vi "AlliGator Compute Phasor Plot's Phasor Ratio.vi"(4 "State Indicators Refnum":refnum<vi>, 5 "Time Stamp Array":dbl[](array[numeric]), 7 "Phasor Graph":refnum<vi>, 8 "Error In":errorcluster, 9 "Plot Idx":i32, 10 "Phasor Ratio Graph":refnum<vi>, 11 "Lifetime Graph":refnum<vi>) -> (0 "Error Out":errorcluster, 1 "Message":string)   [LabVIEW 2021, in "AlliGator Phasor Ratio.lvlib"]
doc: "Computes phasor ratio and derived quantities and outputs the corresponding plots."
uses:
  AlliGator Phasor Ratio.lvlib
  GUI/AlliGator State Indicator.ctl
  Settings/AlliGator Settings List.ctl
  Phasor/Phasor Ratio Type.ctl
  Phasor/Phasor.lvlib
  Globals, Variables, Constants/AlliGator Globals, Variables & Constants.lvlib
  Settings/AlliGator Settings.lvlib
  Graphs/XY Graph/XY Graph Add-Ons.lvlib
  Error/Error.lvlib
  Strings/Strings.lvlib
  Sound/Sound.lvlib
  GUI/AlliGator GUI.lvlib
panel:
  # "see the AlliGator License on the block diagram (Ctrl+E or Window:Show Block Diagram)"
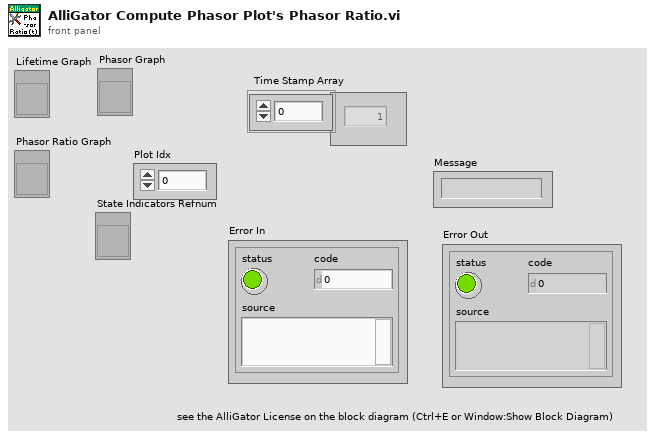
[diagram p1: front panel]
types:
  T1 = typedef "AlliGator State Indicator.ctl" = cluster{"Phasor Calibration Defined":bool, "Phasor Calibration Series Defined":bool, "Phasor Calibration Map Defined":bool, "Phasor Ratio Reference 1 Defined":bool, "Phasor Ratio Reference 2 Defined":bool, "Phasor Ratio Lifetime Reference 1 Defined ":bool, "Phasor Ratio Lifetime Reference 2 Defined":bool, "Phasor Calibration Used":bool, "Phasor Calibration Series Used":bool, "Phasor Calibration Map Used":bool, "Dataset Update Needed":bool, "Phasor Plot Update Needed":bool, "Reference/IRF Defined":bool, "Individual IRFs Defined":bool}
  T2 = typedef "AlliGator Settings.lvlib/AlliGator Settings List.ctl" = enum16{"GUI:Visible Settings Tab", "GUI:Last Run Version", "Source Image:Use Image Histogram for Contrast", "Source Image:Low Count Pixels Rejection Options", "Source Image:High Count Pixels Rejection Options", "Source Image:Use Image Brightness", "Source Image:Blend Overlay with Image Background", "Source Image:Use Fixed ROI Diameter", "Source Image:ROI Diameter", "Source Image:ROI Center Color", "Source Image:Peak Threshold", "Source Image:Intensity Threshold", "Source Image:Image Binning Options", "Source Image:Image Smoothing Options", "Source Image:Image Histogram Active", "Source Image:Invert Binary Mask", "Source Image:Hot Pixel Removal", "Source Image:Overlay Analyzed ROI Center", "Source Image:Auto-Adjust Contrast", "Source Image:Histogram Lower Percentile", "Source Image:Histogram Upper Percentile", "Source Image:Save Source Image", "Source Image:Scale Bar Options", "Source Image:Image Resolution (Pixel Size)", "Source Image:Flatfield Correction", "Source Image:Show Dead Left Columns Correction", "Source Image:Dead Left Columns Correction", "Source Image:Image Pre-Processing Operations Order", "Source Image:Overlay ROI Median", "Source Image:Median Overlay Color", "Data Information:Gate Width", "Data Information:Nanotime Gate Separation", "Data Information:Macrotime Gate Separation", "Data Information:Gate Step", "Data Information:# Gates", "Data Information:Gate Image Exposure", "Data Information:Gate Image Integration", "Data Information:Gates to Skip", "Data Information:Gates to Keep", "Data Information:Define Gates to", "Data Information:Channel Name", "Data Information:Available Channel Names", "Data Information:Channel Arithmetic", "Data Information:Background File Subtraction", "Data Information:Background File", "Data Information:Background Scaling Factor", "Data Information:Background Pile-up Correction", "Data Information:Background Pixel Well Capacity", "Data Information:Laser Period", "Data Information:SYNC Period", "Data Information:Pile-up Correction", "Data Information:Pixel Well Capacity", "Data Information:Dataset Scaling Factor", "Fluorescence Decay_Decay Pre-Processing:Reverse Gates", "Fluorescence Decay_Decay Pre-Processing:Verbose Decay Pre-Processing", "Fluorescence Decay_Decay Pre-Processing:Use Decay Pre-Processing", "Fluorescence Decay_Decay Pre-Processing:Background Subtraction", "Fluorescence Decay_Decay Pre-Processing:Background Definition Range", "Fluorescence Decay_Decay Pre-Processing:Baseline Subtraction Method", "Fluorescence Decay_Decay Pre-Processing:Decay Pre-Processing Operations Order", "Fluorescence Decay_Decay Pre-Processing:Smoothing Parameter", "Fluorescence Decay_Decay Pre-Processing:Shift Decay", "Fluorescence Decay_Decay Pre-Processing:Decay Shift Parameters", "Fluorescence Decay_Decay Pre-Processing:Fold Decay", "Fluorescence Decay_Decay Pre-Processing:# Folds", "Fluorescence Decay_Decay Pre-Processing:1-Normalize Decay", "Fluorescence Decay_Decay Pre-Processing:[0-1]-Normalize Decay", "Fluorescence Decay_Decay Pre-Processing:Smoothen Decay", "Fluorescence Decay_Decay Pre-Processing:Extrapolate Decay", "Fluorescence Decay_Decay Pre-Processing:Use Periodicity", "Fluorescence Decay_Decay Pre-Processing:Use Cursors", "Fluorescence Decay_Decay Pre-Processing:Tail Fraction", "Fluorescence Decay_Decay Pre-Processing:Head Fraction", "Fluorescence Decay_Decay Pre-Processing:Additional Points", "Fluorescence Decay_Decay Pre-Processing:Straighten Decay", "Fluorescence Decay_Decay Pre-Processing:Constant Background", "Fluorescence Decay_Decay Pre-Processing:Pixel-Normalize Decay", "Fluorescence Decay_Advanced Analysis:Extract IRF instead of Decay", "Fluorescence Decay_Advanced Analysis:IRF Extraction Options", "Fluorescence Decay_Advanced Analysis:IRF Optimization Options", "Fluorescence Decay_Advanced Analysis:Square Pulse Options", "Fluorescence Decay_Advanced Analysis:IRF Order", "Fluorescence Decay_Advanced Analysis:IRF Time Constants", "Fluorescence Decay_Advanced Analysis:Wavelet Analysis Options", "Fluorescence Decay_Advanced Analysis:Average Lifetime Options", "Fluorescence Decay_Fit Options:Fit Options", "Fluorescence Decay_Fit Options:Use Legacy Fitting Approach", "Fluorescence Decay_Fit Options:Use Data Information Laser Period", "Fluorescence Decay_Fit Parameters:Displayed Fit Parameters", "Fluorescence Decay_Fit Parameters:Fit Parameter Constraints", "Fluorescence Decay_Fit Parameters:Export Tabulated Results", "Fluorescence Decay_Fit Parameters:MLE Baseline Offset Type", "Fluorescence Decay_Fit Parameters:MLE Baseline Offset", "Fluorescence Decay_Fit Parameters:Guess Parameter Names", "Fluorescence Decay_Fit Parameters:Guess Parameter Values", "Fluorescence Decay_Fit Parameters:Guess Parameters Options", "Fluorescence Decay_Styles:Show Last Decay Only", "Fluorescence Decay_Styles:Decay Graph Color Array", "Fluorescence Decay:Decay Graph Active", "Fluorescence Decay Statistics:Min Peak Value", "Fluorescence Decay Statistics:Reject Low Decay Peak Pixels", "Fluorescence Decay Statistics:Reject High Decay Peak Pixels", "Fluorescence Decay Statistics:Max Peak Value", "Time Traces:Use File Timestamp", "Time Traces:Time Step", "Time Traces:Use Intensity Correction File", "Time Traces:Intensity Correction File", "Phasor Plot:Phasor Plot Smoothing Options", "Phasor Plot:Phasor Plot Size", "Phasor Plot:Phasor Plot Graphics Options", "Phasor Plot:Cumulative Phasor Plot", "Phasor Plot:Use Phasor Brightness", "Phasor Plot:Blend Overlay with Phasor Background", "Phasor Plot:Save Phasor Plot", "Phasor Plot:Show References", "Phasor Plot:Phasor Ratio Decay Range", "Phasor Plot:Exponential Fading", "Phasor Plot:Phasor Ratio Reference Colors", "Phasor Plot:Reference Radius", "Phasor Plot:Show Color Map Vertices", "Phasor Plot:Phasor Plot Active", "Phasor Plot:Phasor Ratio Color Map Type", "Phasor Plot:Phasor Ratio Color Map", "Phasor Plot:Phasor Ratio Display Range", "Phasor Plot:Selected Image ROI(s)", "Phasor Plot:All Image ROIs", "Phasor Plot:Selected Phasor Plot ROI(s)", "Phasor Plot:All Phasor Plot ROIs", "Phasor Plot:Phasor Ratio Color-Coded Quantity", "Phasor Plot:Store Phasor Harmonics", "Phasor Plot:Draw Reference Segment", "Phasor Plot:User-Defined Quantity", "Phasor Graph:Phasor Frequency", "Phasor Graph:Phasor Ratio Type", "Phasor Graph:Pixel-level Phasor Computation", "Phasor Graph:Save Phasor Graph", "Phasor Graph:Phasor Graph Active", "Phasor Graph:Phasor SDV Options", "Phasor Calibration:Use Backup Calibration if needed", "Phasor Graph:Define Shortest Lifetime as", "Phasor Calibration:Backup Calibration Type", "Phasor Calibration:Calibration Type", "Phasor Calibration:Calibration Lifetime", "Phasor Calibration:Calibration Map Algorithm", "Single-Exponential Phasor Locus (SEPL):Gate Parameters", "Single-Exponential Phasor Locus (SEPL):User-defined Gate", "Single-Exponential Phasor Locus (SEPL):User-defined IRF", "Single-Exponential Phasor Locus (SEPL):Phasor Parameters", "Single-Exponential Phasor Locus (SEPL):Decay & IRF Parameters", "Single-Exponential Phasor Locus (SEPL):Display Parameters", "Lifetime Analysis:Decay Analysis Parameters", "Lifetime Analysis:Lifetime Map Active", "Plugins:Python Settings", "Miscellaneous:Verbose Mode", "Miscellaneous:Beep after Script", "Miscellaneous:Saved Image File Format", "Miscellaneous:Exported Gate Image Settings", "Miscellaneous:Include Loading in Timing", "Miscellaneous:Verbose Settings Mode", "Miscellaneous:Histogram Options", "Miscellaneous:Beep on Error", "Miscellaneous:# Logical Processors Used", "Miscellaneous:ROI Description Max Characters", "Miscellaneous:Verbose Error Mode", "Miscellaneous:Transparent Mask Color"}
  T3 = typedef "Phasor.lvlib/Phasor Ratio Type.ctl" = enum32{"Intensity-weighted", "Amplitude-weighted"}
  T4 = typedef "Phasor.lvlib/Phasor (g, s).ctl" = cluster{"g":dbl, "s":dbl}
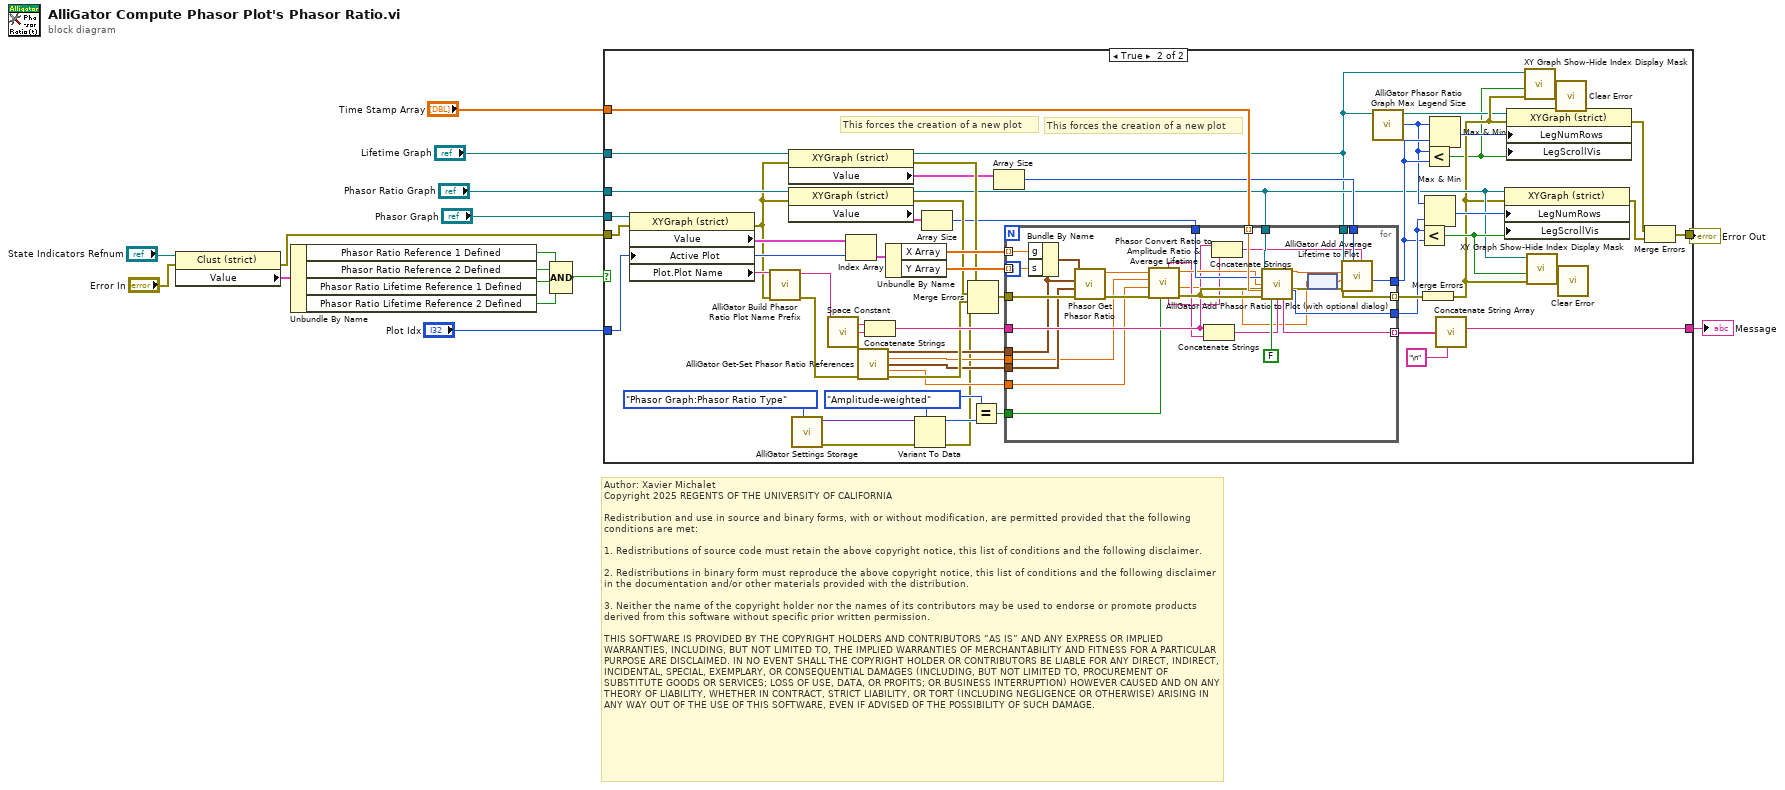
[diagram p0: block diagram]
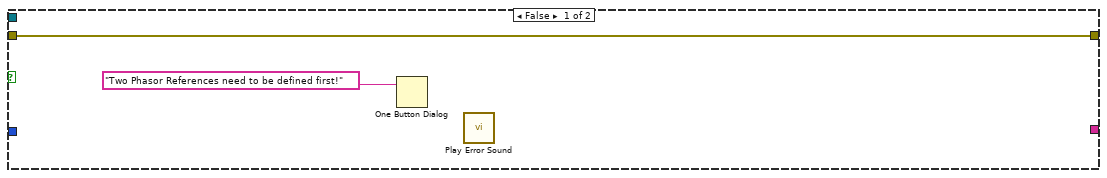
[diagram p2: hidden frame]
diagram:
  # "Author: Xavier Michalet\nCopyright 2025 REGENTS OF THE UNIVERSITY OF CALIFORNIA\n\nRedistribution and use in source and binary forms, with or without modification, are permitted provided that the following conditions are met:\n\n1. Redistributions of source code must retain the above copyright notice, this list of conditions and the following disclaimer.\n\n2. Redistributions in binary form must reproduce the above copyright notice, this list of conditions and the following disclaimer in the documentation and/or other materials provided with the distribution.\n\n3. Neither the name of the copyright holder nor the names of its contributors may be used to endorse or promote products derived from this software without specific prior written permission.\n\nTHIS SOFTWARE IS PROVIDED BY THE COPYRIGHT HOLDERS AND CONTRIBUTORS “AS IS” AND ANY EXPRESS OR IMPLIED WARRANTIES, INCLUDING, BUT NOT LIMITED TO, THE IMPLIED WARRANTIES OF MERCHANTABILITY AND FITNESS FOR A PARTICULAR PURPOSE ARE DISCLAIMED. IN NO EVENT SHALL THE COPYRIGHT HOLDER OR CONTRIBUTORS BE LIABLE FOR ANY DIRECT, INDIRECT, INCIDENTAL, SPECIAL, EXEMPLARY, OR CONSEQUENTIAL DAMAGES (INCLUDING, BUT NOT LIMITED TO, PROCUREMENT OF SUBSTITUTE GOODS OR SERVICES; LOSS OF USE, DATA, OR PROFITS; OR BUSINESS INTERRUPTION) HOWEVER CAUSED AND ON ANY THEORY OF LIABILITY, WHETHER IN CONTRACT, STRICT LIABILITY, OR TORT (INCLUDING NEGLIGENCE OR OTHERWISE) ARISING IN ANY WAY OUT OF THE USE OF THIS SOFTWARE, EVEN IF ADVISED OF THE POSSIBILITY OF SUCH DAMAGE."
  n1 = property class="Clust (strict)"(reference="State Indicators Refnum", error in="Error In") -> (error out=w2:errorcluster, "Value"=w4:T1)  [unwired: 1 out]
  n2 = Unbundle By Name(w4) -> ("Phasor Ratio Reference 1 Defined"=w14:bool, "Phasor Ratio Reference 2 Defined"=w13:bool, "Phasor Ratio Lifetime Reference 1 Defined"=w12:bool, "Phasor Ratio Lifetime Reference 2 Defined"=w11:bool)
  n3 = Compound Arithmetic op=AND(w14, w13, w12, w11) -> (w10:bool)
  n4 = case shown="True" w10 {
    tunnel: "Lifetime Graph" -> [_ w72]
    tunnel: "Phasor Ratio Graph" -> [_ w71]
    tunnel: w2 -> [w17 w69]
    tunnel: [w17 w38] -> w9
    tunnel: "Phasor Graph" -> [_ w70]
    tunnel: "Time Stamp Array" -> [_ w62]
    tunnel: "Plot Idx" -> [_ w51]
    tunnel: [_ w20] -> w1
    frame False {
      n5 = One Button Dialog(message="Two Phasor References need to be defined first!") -> ()  [unwired: 1 in, 1 out]
      n6 = call "Play Error Sound.vi"() -> ()  [unwired: 27 in, 1 out]
    }
    frame True {
      w26 = Phasor_Ratio_Type."Amplitude-weighted" ("Phasor Ratio Type")
      # "This forces the creation of a new plot"
      # "This forces the creation of a new plot"
      n7 = property class="XYGraph (strict)"(reference=w70, error in=w69, "Active Plot"=w51) -> (error out=w45:errorcluster, "Value"=w60:cluster{"X Array":dbl[], "Y Array":dbl[]}[], "Plot.Plot Name"=w50:string)  [unwired: 1 out]
      n8 = call "AlliGator Build Phasor Ratio Plot Name Prefix.vi"("Error In"=w45, "Phasor Plot Name in"=w50) -> ("Error Out"=w44:errorcluster, "Phasor Ratio Plot Name Prefix out"=w49:string)  [unwired: 8 in]
      n9 = property class="XYGraph (strict)"(reference=w72, error in=w45) -> (reference out=w29:refnum<vi>, error out=w65:errorcluster, "Value"=w58:cluster{"X Array":dbl[], "Y Array":dbl[]}[])
      n10 = property class="XYGraph (strict)"(reference=w71, error in=w45) -> (reference out=w32:refnum<vi>, error out=w64:errorcluster, "Value"=w61:cluster{"X Array":dbl[], "Y Array":dbl[]}[])
      n11 = call "AlliGator Settings Storage.vi"("AlliGator Settings List"=AlliGator_Settings_List."Phasor Graph:Phasor Ratio Type") -> ("Error Out"=w24:errorcluster, "Variant Data out"=w25:variant)  [unwired: 9 in]
      n12 = call <vilib>:"Space Constant.vi"() -> ("String"=w47:string)
      n13 = Index Array(array=w60, index=w51) -> (element=w68:cluster{"X Array":dbl[], "Y Array":dbl[]})
      n14 = call "AlliGator Get-Set Phasor Ratio References.vi"("error in (no error)"=w44) -> ("Reference Phasor 1"=w42:T4, "Reference Lifetime 1"=w40:dbl[unit], "Reference Phasor 2"=w41:T4, "Reference Lifetime 2"=w39:dbl[unit], "error out"=w43:errorcluster)  [unwired: 7 in, 3 out]
      n15 = Concatenate Strings(w49, w47) -> (w48:string)
      n16 = Unbundle By Name(w68) -> ("X Array"=w67:dbl[], "Y Array"=w66:dbl[])
      n17 = Variant To Data(error in=w24, type=w26, Variant=w25) -> (data=w27:T3, error out=w22:errorcluster)
      n18 = Array Size(array=w61) -> (size(s)=w59:i32)
      n19 = Merge Errors(w65, w64, w43, w22) -> (w63:errorcluster)
      n20 = Equal?(x=w26, y=w27) -> (x = y?=w23:bool)
      n21 = Array Size(array=w58) -> (size(s)=w57:i32)
      n22 = for {
        tunnel: w29 -> [w103]
        tunnel: w32 -> [w102]
        tunnel: w67 -> [w99] mode=indexing
        tunnel: w66 -> [w98] mode=indexing
        tunnel: w62 -> [w95] mode=indexing
        tunnel: w59 -> [w94]
        tunnel: w57 -> [w93]
        tunnel: [w92] -> w53
        tunnel: [w91] -> w52
        tunnel: w48 -> [w85]
        tunnel: w63 -> [w100]
        tunnel: [w83] -> w56 mode=indexing
        tunnel: w42 -> [w82]
        tunnel: w41 -> [w81]
        tunnel: w40 -> [w79]
        tunnel: w39 -> [w78]
        tunnel: w23 -> [w76]
        tunnel: [w75] -> w21 mode=indexing
        n23 = Bundle By Name(cluster=w82, "g"=w99, "s"=w98) -> (w97:T4)
        n24 = call "Phasor Get Phasor Ratio.vi"("Error In"=w100, "Reference Phasor 2"=w81, "Reference Phasor 1"=w82, "Phasor"=w97) -> ("Error Out"=w89:errorcluster, "Phasor Ratio (f1)"=w90:dbl)  [unwired: 5 in, 1 out]
        n25 = call "Phasor Convert Ratio to Amplitude Ratio & Average Lifetime.vi"("Compute Amplitude Ratio"=w76, "error in (no error)"=w89, "Reference Lifetime 2"=w78, "Reference Lifetime 1"=w79, "Phasor Ratio (f1)"=w90) -> ("error out"=w88:errorcluster, "Average Lifetime"=w74:dbl[unit], "Phasor/Amplitude Ratio"=w87:dbl, "Average Lifetime Caption"=w77:string, "Phasor Ratio Plot Name Suffix"=w80:string)  [unwired: 2 in]
        n26 = Concatenate Strings(w85, w80) -> (w86:string)
        n27 = Concatenate Strings(w85, w77) -> (w84:string)
        n28 = call "AlliGator Add Phasor Ratio to Plot (with optional dialog).vi"("XYGraph in"=w102, "Plot ID (-1)"=w94, "Phasor Ratio"=w87, "Time Point"=w95, "error in (no error)"=w88, "Interactive?"=FALSE, "New Plot Name"=w86) -> ("Sample Abscissa"=w101:dbl, "# Plots"=w92:i32, "Message"=w75:string)  [unwired: 3 in, 3 out]
        n29 = node(w74) -> (w73:dbl)
        n30 = call "AlliGator Add Average Lifetime to Plot.vi"("New Plot Name"=w84, "Plot ID (-1)"=w93, "error in (no error)"=w88, "Average Lifetime"=w73, "Abscissa"=w101, "Lifetime Graph refnum"=w103) -> ("error out"=w83:errorcluster, "# Plots"=w91:i32)  [unwired: 2 in, 2 out]
      }
      n31 = call "AlliGator Phasor Ratio Graph Max Legend Size.vi"() -> ("Phasor Ratio Graph Max Legend Size"=w46:i32)  [unwired: 5 in]
      n32 = Less?(x=w53, y=w52) -> (x < y?=w33:bool)
      n33 = Merge Errors(w56) -> (w30:errorcluster)
      n34 = Less?(x=w46, y=w52) -> (x < y?=w28:bool)
      n35 = Max & Min(x=w46, y=w53) -> (min(x,y)=w54:i32)  [unwired: 1 out]
      n36 = Max & Min(x=w46, y=w52) -> (min(x,y)=w55:i32)  [unwired: 1 out]
      n37 = call "Concatenate String Array.vi"("Separator (TAB)"="\n", "String Array"=w21) -> ("Formatted String"=w20:string)  [unwired: 9 in]
      n38 = property class="XYGraph (strict)"(reference=w32, error in=w30, "LegNumRows"=w54, "LegScrollVis"=w33) -> (error out=w36:errorcluster)  [unwired: 1 out]
      n39 = property class="XYGraph (strict)"(reference=w29, error in=w30, "LegNumRows"=w55, "LegScrollVis"=w28) -> (error out=w37:errorcluster)  [unwired: 1 out]
      n40 = call "XY Graph Show-Hide Index Display Mask.vi"("error in (no error)"=w30, "Show(T)/Hide(F)"=w28, "XYGraph Ref"=w29) -> ("error out"=w31:errorcluster)  [unwired: 7 in, 1 out]
      n41 = call "XY Graph Show-Hide Index Display Mask.vi"("error in (no error)"=w30, "Show(T)/Hide(F)"=w33, "XYGraph Ref"=w32) -> ("error out"=w34:errorcluster)  [unwired: 7 in, 1 out]
      n42 = call "Clear Error.vi"("Error In"=w31) -> ()  [unwired: 8 in, 1 out]
      n43 = call "Clear Error.vi"("Error In"=w34) -> ()  [unwired: 8 in, 1 out]
      n44 = Merge Errors(w37, w36) -> (w38:errorcluster)
    }
  }
  "Error Out" <- w9
  "Message" <- w1
